vi "XML-RPC Request Parser.vi"(8 "error in (no error)":errorcluster, 11 "XML-RPC Call":string="POST /xmlrpc HTTP/1.1\r\nContent-Type: text/xml\r\nUser-Agent: Apache XML RPC 3.0 (Jakarta Commons httpclient Transport)\r\nHost: s881643.srn.sandia.gov:8080\r\nContent-Length: 162\r\n\r\n<?xml version=\"1.0\" encoding=\"UTF-8\"?><methodCall><methodName>Dialog Test.vi</methodName><params><param><value>mystringparam</value></param></params></methodCall>") -> (0 "error out":errorcluster, 2 "Parameters":string[](array[string]), 3 "methodName":string)   [LabVIEW 2014]
doc: "Unpack XML-RPC method request parameters into an array of XML-RPC formatted values"
panel:
  in  "XML-RPC Validation for  Method Call":string="<\\?xml version=\"1.0\".*\\?>[\\s\\n\\r\\t]*<methodCall>[\\s\\n\\r\\t]*<methodName>.*</methodName>.*</methodCall>"
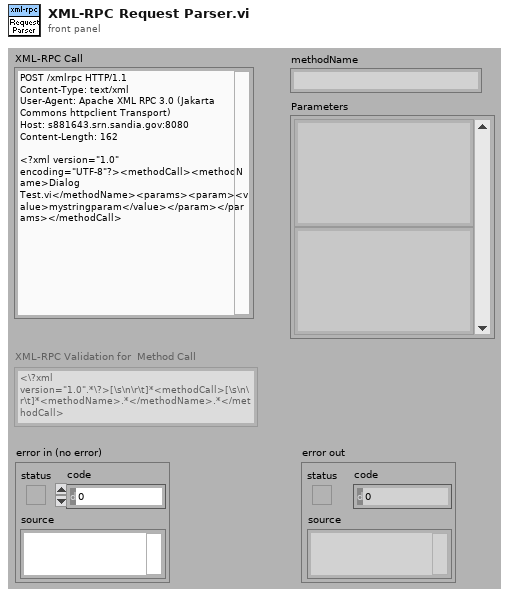
[diagram p1: front panel]
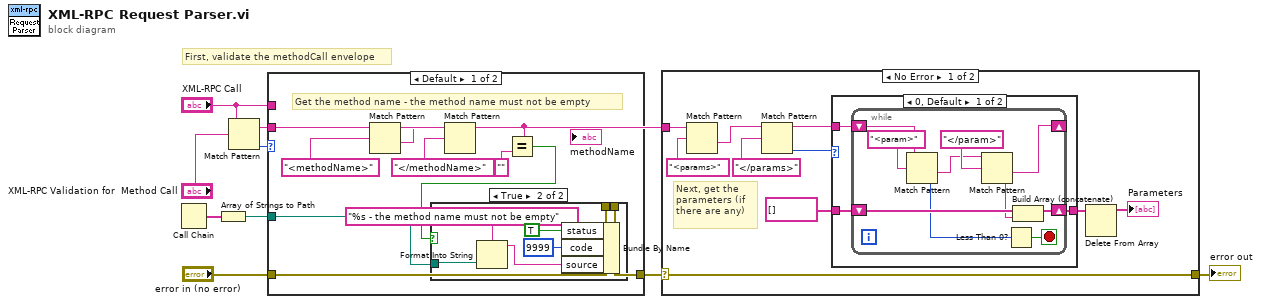
[diagram p0: block diagram]
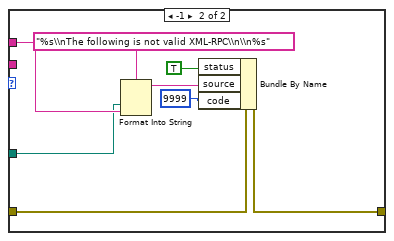
[diagram p5: hidden frame]
diagram:
  # "First, validate the methodCall envelope"
  n1 = Call Chain() -> (call chain=w5:string[])
  n2 = Array of Strings to Path(0:w5) -> (2:w4:path)  [unwired: 1 in]
  n3 = Match Pattern(string="XML-RPC Call", regular expression="XML-RPC Validation for  Method Call") -> (match substring=w1:string, offset past match=w8:i32)  [unwired: 1 in, 2 out]
  n4 = case shown="Default" w8 {
    tunnel: "error in (no error)" -> [w13 w35]
    tunnel: [w12 w34] -> w3
    tunnel: "XML-RPC Call" -> [_ w29]
    tunnel: w1 -> [w19 _]
    tunnel: w4 -> [w11 w28]
    frame Default {
      # "Get the method name - the method name must not be empty"
      n5 = Match Pattern(string=w19, regular expression="<methodName>") -> (after substring=w16:string)  [unwired: 1 in, 3 out]
      n6 = Match Pattern(string=w16, regular expression="</methodName>") -> (before substring=w15:string)  [unwired: 1 in, 3 out]
      "methodName" <- w15
      n7 = Equal?(x=w15, y="") -> (x = y?=w10:bool)
      n8 = case shown="True" w10 {
        tunnel: w13 -> [w20 w27]
        tunnel: w11 -> [_ w26]
        tunnel: [w20 w22] -> w12
        frame False {
        }
        frame True {
          n9 = Format Into String(format string="%s - the method name must not be empty", w26) -> (resulting string=w25:string)  [unwired: 2 in, 1 out]
          n10 = Bundle By Name(cluster=w27, "status"=TRUE, "code"=9999, "source"=w25) -> (w22:errorcluster)
        }
      }
    }
    frame -1 {
      n11 = Format Into String(format string="%s\\nThe following is not valid XML-RPC\\n\\n%s", w28, w29) -> (resulting string=w31:string)  [unwired: 2 in, 1 out]
      n12 = Bundle By Name(cluster=w35, "status"=TRUE, "source"=w31, "code"=9999) -> (w34:errorcluster)
    }
  }
  n13 = case shown="No Error" w3 {
    selector: w3 -> [w45 w60]
    tunnel: [w45 w60] -> w2
    tunnel: w1 -> [w42 _]
    frame No Error {
      # "Next, get the parameters (if there are any)"
      n14 = Match Pattern(string=w42, regular expression="<params>") -> (after substring=w44:string)  [unwired: 1 in, 3 out]
      n15 = Match Pattern(string=w44, regular expression="</params>") -> (before substring=w39:string, offset past match=w40:i32)  [unwired: 1 in, 2 out]
      n16 = case shown="0, Default" w40 {
        tunnel: w39 -> [w48 _]
        tunnel: string[] [] -> [w47 w59]
        tunnel: [w46 w59] -> w37
        frame 0, Default {
          n17 = while {
            shift-right: [w54] -> _
            shift-left: w48 -> [w56]
            shift-right: [w51] -> w46
            shift-left: w47 -> [w53]
            stop <- w50 stop-if-true
            n18 = Match Pattern(string=w56, regular expression="<param>") -> (after substring=w57:string, offset past match=w49:i32)  [unwired: 1 in, 2 out]
            n19 = Match Pattern(string=w57, regular expression="</param>") -> (before substring=w52:string, after substring=w54:string)  [unwired: 1 in, 2 out]
            n20 = Less Than 0?(x=w49) -> (x < 0?=w50:bool)
            n21 = Build Array (concatenate)(w53, w52) -> (w51:string[])
          }
        }
        frame -1 {
          # "This call doesn't have any parameters"
        }
      }
      n22 = Delete From Array(array=w37) -> (array with subset deleted=→"Parameters":string[])  [unwired: 2 in, 1 out]
    }
    frame Error {
    }
  }
  "error out" <- w2
